vi "LSMcontroller_v66_improvedwfhandling.vi"() -> ()   [LabVIEW 2015] (continued)
                    n3096 = property on="finite samples" class="Bool (strict)"("Value"=w6474) -> ()  [unwired: 2 in, 2 out]
                    n3097 = property on="wavdet" class="Bool (strict)"("Value"=w6474) -> ()  [unwired: 2 in, 2 out]
                    n3098 = property on="save\ndata" class="Bool (strict)"("Value"=w6474) -> ()  [unwired: 2 in, 2 out]
                    n3099 = local write "Save tab"(enum32{"withsave", "withoutsave"}."withsave" ("Save tab")) -> ()
                    n3100 = property on="# of frames" class="DigNum (strict)"("DisabledEnum"=T7."Disabled and Grayed Out" ("Disabled")) -> ()  [unwired: 2 in, 2 out]
                    n3101 = property on="save\ndata" class="Bool (strict)"("DisabledEnum"=T7."Disabled and Grayed Out" ("Disabled")) -> ()  [unwired: 2 in, 2 out]
                  }
                }
              }
              frame #1 {
                n3102 = local read "finite samples"() -> (w6484:bool)
                n3103 = local read "continuous"() -> (w6483:bool)
                n3104 = local read "wavdet"() -> (w6482:bool)
                n3105 = call "2pparameters.vi"("command"="get") -> ("params out"=w6478:T10)  [unwired: 1 in]
                n3106 = Bundle By Name(cluster=w6478, "finite"=w6484, "cont"=w6483, "wavdet"=w6482) -> (w6481:T10)
                n3107 = call "2pparameters.vi"("Params in"=w6481, "command"="set") -> ()  [unwired: 1 out]
              }
            }
          }
          event "wavdet": Value Change {
            n3108 = event-data() -> ("NewVal"=w6485:bool)  [unwired: 1 in]
            n3109 = flat-sequence {
              tunnel: w6485 -> [w6486]
              frame #0 {
                n3110 = case shown="False" w6486 {
                  frame False {
                    n3111 = property on="finite samples" class="Bool (strict)"("Value"=TRUE ("finite samples for recording")) -> ()  [unwired: 2 in, 2 out]
                    n3112 = property on="continuous" class="Bool (strict)"("Value"=FALSE ("continuous")) -> ()  [unwired: 2 in, 2 out]
                    n3113 = local write "Save tab"(enum32{"withsave", "withoutsave"}."withsave" ("Save tab")) -> ()
                    n3114 = property on="save\ndata" class="Bool (strict)"("DisabledEnum"=T7."Enabled" ("Disabled")) -> ()  [unwired: 2 in, 2 out]
                    n3115 = property on="# of frames" class="DigNum (strict)"("DisabledEnum"=T7."Enabled" ("Disabled")) -> ()  [unwired: 2 in, 2 out]
                    n3116 = property on="save\ndata" class="Bool (strict)"("Value"=TRUE ("save\ndata")) -> ()  [unwired: 2 in, 2 out]
                  }
                  frame True {
                    w6495 = FALSE ("finite samples for recording")
                    n3117 = property on="finite samples" class="Bool (strict)"("Value"=w6495) -> ()  [unwired: 2 in, 2 out]
                    n3118 = property on="continuous" class="Bool (strict)"("Value"=w6495) -> ()  [unwired: 2 in, 2 out]
                    n3119 = property on="save\ndata" class="Bool (strict)"("DisabledEnum"=T7."Enabled" ("Disabled")) -> ()  [unwired: 2 in, 2 out]
                    n3120 = local write "Save tab"(enum32{"withsave", "withoutsave"}."withsave" ("Save tab")) -> ()
                    n3121 = property on="# of frames" class="DigNum (strict)"("DisabledEnum"=T7."Disabled" ("Disabled")) -> ()  [unwired: 2 in, 2 out]
                    n3122 = property on="save\ndata" class="Bool (strict)"("Value"=TRUE ("save\ndata")) -> ()  [unwired: 2 in, 2 out]
                  }
                }
              }
              frame #1 {
                n3123 = local read "finite samples"() -> (w6498:bool)
                n3124 = local read "continuous"() -> (w6499:bool)
                n3125 = local read "wavdet"() -> (w6500:bool)
                n3126 = call "2pparameters.vi"("command"="get") -> ("params out"=w6504:T10)  [unwired: 1 in]
                n3127 = Bundle By Name(cluster=w6504, "finite"=w6498, "cont"=w6499, "wavdet"=w6500) -> (w6501:T10)
                n3128 = call "2pparameters.vi"("Params in"=w6501, "command"="set") -> ()  [unwired: 1 out]
              }
            }
          }
          event "cursors": Value Change {
            n3129 = event-data() -> ()  [unwired: 1 in, 5 out]
            n3130 = case shown="True" "cursors" {
              frame False {
                n3131 = property on="img_CH1" class="IntGraph (strict)"("Active Cursor"=u32 0, "Cursor.Cursor Style"=u8 0 ("Cursor Style"), "Cursor.Cursor Point Style"=u8 0 ("Cursor Point Style")) -> ("Cursor.Cursor Position:Cursor X"=w6509:dbl, "Cursor.Cursor Position:Cursor Y"=w6510:dbl)  [unwired: 2 in, 2 out]
                n3132 = property on="img_CH2" class="IntGraph (strict)"("Active Cursor"=u32 0, "Cursor.Cursor Style"=u8 0 ("Cursor Style"), "Cursor.Cursor Point Style"=u8 0 ("Cursor Point Style")) -> ()  [unwired: 2 in, 2 out]
                n3133 = local write "cursor x [pixel]"(w6509) -> ()
                n3134 = local write "cursor y [pixel]"(w6510) -> ()
              }
              frame True {
                n3135 = stacked-sequence {
                  frame #0 {
                    n3136 = call "2pparameters.vi"("command"="get") -> ("params out"=w6525:T10)  [unwired: 1 in]
                    n3137 = Unbundle By Name(w6525) -> ("Xpixels Img"=w6526:i32, "Ypixels Img"=w6523:i32)
                    n3138 = To Double Precision Float(number=w6523) -> (double precision float=w6517:dbl)
                    n3139 = To Double Precision Float(number=w6526) -> (double precision float=w6522:dbl)
                    n3140 = Divide(x=w6517, y=2.0) -> (x/y=w6518:dbl)
                    n3141 = Divide(x=w6522, y=2.0) -> (x/y=w6520:dbl)
                    n3142 = Round To Nearest(number=w6518) -> (nearest integer value=w6516:dbl)
                    n3143 = Round To Nearest(number=w6520) -> (nearest integer value=w6519:dbl)
                    n3144 = property on="img_CH1" class="IntGraph (strict)"("Active Cursor"=u32 0, "Cursor.Cursor Style"=u8 8 ("Cursor Style"), "Cursor.Cursor Point Style"=u8 5 ("Cursor Point Style"), "Cursor.Cursor Position:Cursor X"=w6519, "Cursor.Cursor Position:Cursor Y"=w6516, "Cursor.Visible"=TRUE) -> ()  [unwired: 2 in, 2 out]
                  }
                  frame #1 {
                    n3145 = call "2pparameters.vi"("command"="get") -> ("params out"=w6545:T10)  [unwired: 1 in]
                    n3146 = call "2pparameters.vi"("command"="get") -> ("params out"=w6543:T10)  [unwired: 1 in]
                    n3147 = property on="img_CH1" class="IntGraph (strict)"("Active Cursor"=u32 0, "Cursor.Cursor Style"=u8 8 ("Cursor Style"), "Cursor.Cursor Point Style"=u8 5 ("Cursor Point Style")) -> ("Cursor.Cursor Position:Cursor X"=w6538:dbl, "Cursor.Cursor Position:Cursor Y"=w6537:dbl, "Cursor.Cursor Index"=w6560:i32, "Cursor.Cursor Plot"=w6559:i32, "Cursor.Visible"=w6530:bool)  [unwired: 2 in, 2 out]
                    "cursor x [pixel]" <- w6538
                    "cursor y [pixel]" <- w6537
                    n3148 = Unbundle By Name(w6545) -> ("Vy-max Img"=w6547:dbl, "Vy-min Img"=w6534:dbl, "Ypixels Img"=w6549:i32)
                    n3149 = Unbundle By Name(w6543) -> ("VX-max Img"=w6544:dbl, "Vx-min Img"=w6532:dbl, "Xpixels Img"=w6548:i32)
                    n3150 = Subtract(x=w6547, y=w6534) -> (x-y=w6552:dbl)
                    n3151 = Subtract(x=w6544, y=w6532) -> (x-y=w6550:dbl)
                    n3152 = local read "img_CH2"() -> (w6556:sgl[][])
                    n3153 = To Double Precision Float(number=w6548) -> (double precision float=w6551:dbl)
                    n3154 = local read "img_CH1"() -> (w6557:sgl[][])
                    n3155 = To Double Precision Float(number=w6549) -> (double precision float=w6553:dbl)
                    n3156 = Index Array(array=w6557, index (row)=w6560, index (col)=w6559) -> (element=→"value CH 1":sgl)
                    n3157 = Index Array(array=w6556, index (row)=w6560, index (col)=w6559) -> (element=→"value CH 2":sgl)
                    n3158 = Divide(x=w6550, y=w6551) -> (x/y=w6554:dbl)
                    n3159 = Divide(x=w6552, y=w6553) -> (x/y=w6555:dbl)
                    n3160 = Multiply(x=w6538, y=w6554) -> (x*y=w6533:dbl)
                    n3161 = Multiply(x=w6537, y=w6555) -> (x*y=w6536:dbl)
                    n3162 = property on="img_CH2" class="IntGraph (strict)"("Active Cursor"=u32 0, "Cursor.Cursor Style"=u8 8 ("Cursor Style"), "Cursor.Cursor Point Style"=u8 5 ("Cursor Point Style"), "Cursor.Cursor Position:Cursor X"=w6538, "Cursor.Cursor Position:Cursor Y"=w6537, "Cursor.Visible"=w6530) -> ()  [unwired: 2 in, 2 out]
                    n3163 = Add(x=w6533, y=w6532) -> (x+y=w6531:dbl)
                    n3164 = Add(x=w6536, y=w6534) -> (x+y=w6535:dbl)
                    n3165 = local write "Vx-ref"(w6531) -> ()
                    n3166 = local write "Vy-ref"(w6535) -> ()
                  }
                }
              }
            }
          }
          event "img_CH1": Cursor Move {
            n3167 = event-data() -> ("CursIdx"=w6565:i32)  [unwired: 1 in]
            n3168 = Equal To 0?(x=w6565) -> (x = 0?=w6566:bool)
            n3169 = case shown="True" w6566 {
              frame False {
              }
              frame True {
                n3170 = call "2pparameters.vi"("command"="get") -> ("params out"=w6586:T10)  [unwired: 1 in]
                n3171 = call "2pparameters.vi"("command"="get") -> ("params out"=w6588:T10)  [unwired: 1 in]
                n3172 = property on="img_CH1" class="IntGraph (strict)"("Active Cursor"=u32 0, "Cursor.Cursor Style"=u8 8 ("Cursor Style"), "Cursor.Cursor Point Style"=u8 5 ("Cursor Point Style")) -> ("Cursor.Cursor Position:Cursor X"=w6575:dbl, "Cursor.Cursor Position:Cursor Y"=w6574:dbl, "Cursor.Cursor Plot"=w6594:i32, "Cursor.Cursor Index"=w6593:i32, "Cursor.Visible"=w6567:bool)  [unwired: 2 in, 2 out]
                n3173 = Unbundle By Name(w6586) -> ("Vy-max Img"=w6584:dbl, "Vy-min Img"=w6573:dbl, "Ypixels Img"=w6582:i32)
                n3174 = Unbundle By Name(w6588) -> ("VX-max Img"=w6587:dbl, "Vx-min Img"=w6568:dbl, "Xpixels Img"=w6583:i32)
                n3175 = Subtract(x=w6584, y=w6573) -> (x-y=w6579:dbl)
                n3176 = Subtract(x=w6587, y=w6568) -> (x-y=w6581:dbl)
                n3177 = local write "cursor x [pixel]"(w6575) -> ()
                n3178 = local write "cursor y [pixel]"(w6574) -> ()
                n3179 = To Double Precision Float(number=w6583) -> (double precision float=w6580:dbl)
                n3180 = To Double Precision Float(number=w6582) -> (double precision float=w6578:dbl)
                n3181 = local read "img_CH2"() -> (w6595:sgl[][])
                n3182 = local read "img_CH1"() -> (w6598:sgl[][])
                n3183 = Index Array(array=w6595, index (row)=w6594, index (col)=w6593) -> (element=w6596:sgl)
                n3184 = Index Array(array=w6598, index (row)=w6594, index (col)=w6593) -> (element=w6597:sgl)
                n3185 = Divide(x=w6581, y=w6580) -> (x/y=w6577:dbl)
                n3186 = Divide(x=w6579, y=w6578) -> (x/y=w6576:dbl)
                n3187 = local write "value CH 2"(w6596) -> ()
                n3188 = Multiply(x=w6575, y=w6577) -> (x*y=w6570:dbl)
                n3189 = local write "value CH 1"(w6597) -> ()
                n3190 = Multiply(x=w6574, y=w6576) -> (x*y=w6572:dbl)
                n3191 = Add(x=w6570, y=w6568) -> (x+y=w6569:dbl)
                n3192 = local write "Vx-ref"(w6569) -> ()
                n3193 = Add(x=w6572, y=w6573) -> (x+y=w6571:dbl)
                n3194 = property on="img_CH2" class="IntGraph (strict)"("Active Cursor"=u32 0, "Cursor.Cursor Style"=u8 8 ("Cursor Style"), "Cursor.Cursor Point Style"=u8 5 ("Cursor Point Style"), "Cursor.Cursor Position:Cursor X"=w6575, "Cursor.Cursor Position:Cursor Y"=w6574, "Cursor.Visible"=w6567) -> ()  [unwired: 2 in, 2 out]
                n3195 = local write "Vy-ref"(w6571) -> ()
              }
            }
          }
          event "img_CH2": Cursor Move {
            n3196 = event-data() -> ("CursIdx"=w6602:i32)  [unwired: 1 in]
            n3197 = Equal To 0?(x=w6602) -> (x = 0?=w6603:bool)
            n3198 = case shown="True" w6603 {
              frame False {
              }
              frame True {
                n3199 = property on="img_CH2" class="IntGraph (strict)"("Active Cursor"=u32 0, "Cursor.Cursor Style"=u8 8 ("Cursor Style"), "Cursor.Cursor Point Style"=u8 5 ("Cursor Point Style")) -> ("Cursor.Cursor Position:Cursor X"=w6611:dbl, "Cursor.Cursor Position:Cursor Y"=w6612:dbl, "Cursor.Cursor Plot"=w6631:i32, "Cursor.Cursor Index"=w6630:i32, "Cursor.Visible"=w6604:bool)  [unwired: 2 in, 2 out]
                n3200 = call "2pparameters.vi"("command"="get") -> ("params out"=w6623:T10)  [unwired: 1 in]
                n3201 = call "2pparameters.vi"("command"="get") -> ("params out"=w6625:T10)  [unwired: 1 in]
                n3202 = local read "img_CH1"() -> (w6635:sgl[][])
                n3203 = local read "img_CH2"() -> (w6632:sgl[][])
                n3204 = local write "cursor x [pixel]"(w6611) -> ()
                n3205 = local write "cursor y [pixel]"(w6612) -> ()
                n3206 = Unbundle By Name(w6623) -> ("Vy-max Img"=w6621:dbl, "Vy-min Img"=w6606:dbl, "Ypixels Img"=w6619:i32)
                n3207 = Unbundle By Name(w6625) -> ("VX-max Img"=w6624:dbl, "Vx-min Img"=w6609:dbl, "Xpixels Img"=w6620:i32)
                n3208 = Index Array(array=w6635, index (row)=w6631, index (col)=w6630) -> (element=w6634:sgl)
                n3209 = Index Array(array=w6632, index (row)=w6631, index (col)=w6630) -> (element=w6633:sgl)
                n3210 = local write "value CH 2"(w6633) -> ()
                n3211 = local write "value CH 1"(w6634) -> ()
                n3212 = Subtract(x=w6621, y=w6606) -> (x-y=w6616:dbl)
                n3213 = Subtract(x=w6624, y=w6609) -> (x-y=w6618:dbl)
                n3214 = To Double Precision Float(number=w6620) -> (double precision float=w6617:dbl)
                n3215 = To Double Precision Float(number=w6619) -> (double precision float=w6615:dbl)
                n3216 = Divide(x=w6618, y=w6617) -> (x/y=w6614:dbl)
                n3217 = Divide(x=w6616, y=w6615) -> (x/y=w6613:dbl)
                n3218 = Multiply(x=w6611, y=w6614) -> (x*y=w6610:dbl)
                n3219 = Multiply(x=w6612, y=w6613) -> (x*y=w6607:dbl)
                n3220 = property on="img_CH1" class="IntGraph (strict)"("Active Cursor"=u32 0, "Cursor.Cursor Style"=u8 8 ("Cursor Style"), "Cursor.Cursor Point Style"=u8 5 ("Cursor Point Style"), "Cursor.Cursor Position:Cursor X"=w6611, "Cursor.Cursor Position:Cursor Y"=w6612, "Cursor.Visible"=w6604) -> ()  [unwired: 2 in, 2 out]
                n3221 = Add(x=w6610, y=w6609) -> (x+y=→"Vx-ref":dbl)
                n3222 = Add(x=w6607, y=w6606) -> (x+y=→"Vy-ref":dbl)
              }
            }
          }
          event "Focus": Value Change {
            n3223 = event-data() -> ()  [unwired: 1 in, 6 out]
            n3224 = flat-sequence {
              frame #0 {
                n3225 = local read "Focus"() -> (w6639:bool)
                n3226 = case shown="True" w6639 {
                  frame False {
                  }
                  frame True {
                    n3227 = local read "Vx-ref"() -> (w6643:dbl)
                    n3228 = local read "Vy-ref"() -> (w6642:dbl)
                    n3229 = local read "zV"() -> (w6640:dbl)
                    n3230 = call "focusvi.vi"("zc"=w6640, "yc"=w6642, "xc"=w6643) -> ("finalz"=→"zV":dbl)
                  }
                }
              }
              frame #1 {
                n3231 = local write "Focus"(FALSE ("Focus")) -> ()
              }
            }
          }
          event "auto shutter": Value Change {
            n3232 = event-data() -> ()  [unwired: 1 in, 6 out]
            n3233 = call "2pparameters.vi"("command"="get") -> ("params out"=w6647:T10)  [unwired: 1 in]
            n3234 = in-place {
              n3235 = in-place-cluster #46(w6647) -> ()  [unwired: 1 out]
              n3236 = local read "auto shutter"() -> (w6649:bool)
              n3237 = in-place-cluster #46("autoshutter"=w6649) -> (w6645:T10)
            }
            n3238 = call "2pparameters.vi"("Params in"=w6645, "command"="set") -> ()  [unwired: 1 out]
          }
          event "auto OD": Value Change {
            n3239 = event-data() -> ()  [unwired: 1 in, 6 out]
            n3240 = call "2pparameters.vi"("command"="get") -> ("params out"=w6652:T10)  [unwired: 1 in]
            n3241 = in-place {
              n3242 = in-place-cluster #47(w6652) -> ()  [unwired: 1 out]
              n3243 = local read "auto OD"() -> (w6654:bool)
              n3244 = in-place-cluster #47("auto OD"=w6654) -> (w6650:T10)
            }
            n3245 = call "2pparameters.vi"("Params in"=w6650, "command"="set") -> ()  [unwired: 1 out]
          }
          event "ODfilt": Value Change {
            n3246 = event-data() -> ("OldVal"=w6655:u16)  [unwired: 1 in, 5 out]
            n3247 = local read "ODfilt"() -> (w6656:u16)
            n3248 = call "2pparameters.vi"("command"="get") -> ("params out"=w6659:T10)  [unwired: 1 in]
            n3249 = call "filterwheelcontrol_nothorlabslib.vi"("Current OD filt"=w6655, "New ODfilt"=w6656) -> ()  [unwired: 1 in]
            n3250 = in-place {
              in-place-border: w6656 -> [w6661]
              n3251 = in-place-cluster #48(w6659) -> ()  [unwired: 1 out]
              n3252 = in-place-cluster #48("ODfilt"=w6661) -> (w6657:T10)
            }
            n3253 = call "2pparameters.vi"("Params in"=w6657, "command"="set") -> ()  [unwired: 1 out]
          }
          event "Exit": Value Change {
            n3254 = event-data() -> ()  [unwired: 1 in, 5 out]
          }
        }
        n3255 = Wait (ms)(milliseconds to wait=u32 50) -> ()  [unwired: 1 out]
      }
      n3256 = while {
        stop <- w69 stop-if-true
        # "Waveform generation"
        n3257 = event shown="[9] \"load changed AOsq\": Value Change" {
          selector: _ -> [_ _ _ _ _ _ _ _ _ _ _ _ _ _ _ _ _ _ _ _ _ _]
          dyn-events: _ -> [_ _ _ _ _ _ _ _ _ _ _ _ _ _ _ _ _ _ _ _ _ _]
          timeout: _ -> [_ _ _ _ _ _ _ _ _ _ _ _ _ _ _ _ _ _ _ _ _ _]
          tunnel: [_ _ _ _ _ _ _ _ _ _ _ _ _ _ _ _ _ _ _ _ _ w2239] -> w69
          event Timeout {
            n3258 = event-data() -> ()  [unwired: 1 in, 3 out]
          }
          event "Add AO wave": Value Change {
            n3259 = event-data() -> ("NewVal"=w70:bool)  [unwired: 1 in, 5 out]
            n3260 = case shown="True" w70 {
              frame False {
              }
              frame True {
                n3261 = stacked-sequence {
                  seq-local: [_ _ w177 _ _ _ _ _] -> [_ _ _ w209 w220 w228 w294 w326]
                  frame #0 {
                    n3262 = local read "Measurement"() -> (w71:T4)
                    n3263 = case shown="\"Timetrace\"" w71 {
                      frame "X-Y-t movie", Default {
                        n3264 = local read "avpp"() -> (w92:i32)
                        n3265 = local read "Angle ref"() -> (w91:dbl)
                        n3266 = local read "ROI Type"() -> (w90:u16)
                        n3267 = local read "xpixels ref"() -> (w87:i32)
                        n3268 = local read "Vx-min ref"() -> (w86:dbl)
                        n3269 = local read "Vx-max ref"() -> (w85:dbl)
                        n3270 = local read "ypixels ref"() -> (w83:i32)
                        n3271 = local read "Vy-min ref"() -> (w84:dbl)
                        n3272 = local read "Vy-max ref"() -> (w80:dbl)
                        n3273 = local read "Sampling rate"() -> (w74:dbl)
                        n3274 = local read "finite samples"() -> (w75:bool)
                        n3275 = local read "continuous"() -> (w78:bool)
                        n3276 = local read "wavdet"() -> (w79:bool)
                        n3277 = local read "# of frames"() -> (w77:i32)
                        n3278 = local read "maxbufferAI"() -> (w76:i32)
                        n3279 = local read "Override AI buffer"() -> (w72:bool)
                        n3280 = call "2pparameters.vi"("command"="get") -> ("params out"=w89:T10)  [unwired: 1 in]
                        n3281 = Bundle By Name(cluster=w89, "type"="X-Y-t movie", "avpp"=w92, "Angle Img"=w91, "Xpixels Img"=w87, "Vx-min Img"=w86, "VX-max Img"=w85, "Ypixels Img"=w83, "Vy-min Img"=w84, "Vy-max Img"=w80, "srate"=w74, "srate Img"=w74, "finite"=w75, "cont"=w78, "wavdet"=w79, "measpoints"=w77, "maxbufferAI"=w76, "Drawing Mode"=w90, "Vz-reset"=0.0, "AIoverride"=w72) -> (w81:T10)
                        n3282 = call "2pparameters.vi"("Params in"=w81, "command"="set") -> ()  [unwired: 1 out]
                      }
                      frame "X-Y-Z stack" {
                        n3283 = call "2pparameters.vi"("command"="get") -> ("params out"=w96:T10)  [unwired: 1 in]
                        n3284 = Bundle By Name(cluster=w96, "type"="X-Y-Z stack") -> (w94:T10)
                        n3285 = call "2pparameters.vi"("Params in"=w94, "command"="set") -> ()  [unwired: 1 out]
                      }
                      frame "Lifetime (scan)" {
                        n3286 = call "2pparameters.vi"("command"="get") -> ("params out"=w101:T10)  [unwired: 1 in]
                        n3287 = Bundle By Name(cluster=w101, "type"="Lifetime (scan)") -> (w99:T10)
                        n3288 = call "2pparameters.vi"("Params in"=w99, "command"="set") -> ()  [unwired: 1 out]
                      }
                      frame "Lifetime (contour)" {
                        n3289 = local read "Vy-min draw"() -> (w111:dbl)
                        n3290 = local read "Vy-max draw"() -> (w110:dbl)
                        n3291 = local read "Vx-min draw"() -> (w113:dbl)
                        n3292 = local read "Vx-max draw"() -> (w112:dbl)
                        n3293 = local read "xpixels ref"() -> (w109:i32)
                        n3294 = local read "ypixels ref"() -> (w108:i32)
                        n3295 = local read "ROI Type"() -> (w107:u16)
                        n3296 = local read "srateAODOtt"() -> (w118:dbl)
                        n3297 = local read "# of frames"() -> (w123:i32)
                        n3298 = local read "refreshtime"() -> (w115:dbl)
                        n3299 = local read "Pel"() -> (w106:dbl)
                        n3300 = local read "bin"() -> (w121:dbl)
                        n3301 = local read "Override AI buffer"() -> (w104:bool)
                        n3302 = local read "finite samples"() -> (w130:bool)
                        n3303 = local read "srateAODOtt"() -> (w117:dbl)
                        n3304 = local read "srateAODOtt"() -> (w124:dbl)
                        n3305 = local read "continuous"() -> (w129:bool)
                        n3306 = local read "Angle ref"() -> (w114:dbl)
                        n3307 = local read "wavdet"() -> (w131:bool)
                        n3308 = local read "Vx-ref"() -> (w126:dbl)
                        n3309 = local read "Vy-ref"() -> (w128:dbl)
                        n3310 = local read "avpp"() -> (w127:i32)
                        n3311 = call "tt_timeandsamples.vi"("bin"=w121, "refreshtime"=w115, "srateAODOtt"=w118, "tot#ofsamples"=w123) -> ("refreshrate"=w119:dbl, "refreshbuffer"=w120:i32, "timetracecycles"=w125:i32)  [unwired: 5 in]
                        n3312 = local read "bin"() -> (w122:dbl)
                        n3313 = call "2pparameters.vi"("command"="get") -> ("params out"=w134:T10)  [unwired: 1 in]
                        n3314 = Bundle By Name(cluster=w134, "Drawing Mode"=w107, "measpoints"=w123, "tt_cycles"=w125, "refreshbuffer"=w120, "refreshrate"=w119, "Vx-ref"=w126, "Vy-ref"=w128, "srate"=w117, "finite"=w130, "cont"=w129, "wavdet"=w131, "avpp"=w127, "srateAODO"=w124, "bufferAI"=w120, "bin"=w122, "Angle Img"=w114, "Vxminref"=w113, "Vxmaxref"=w112, "Vyminref"=w111, "Vymaxref"=w110, "Xpixels Img"=w109, "Ypixels Img"=w108, "Pel"=w106, "Vz-reset"=0.0, "AIoverride"=w104, "type"="Lifetime (contour)") -> (w132:T10)
                        n3315 = Reciprocal(x=w119) -> (1/x=w116:dbl)
                        n3316 = local write "refreshtime"(w116) -> ()
                        n3317 = call "2pparameters.vi"("Params in"=w132, "command"="set") -> ()  [unwired: 1 out]
                      }
                      frame "X-Y-Z-t movie" {
                      }
                      frame "linescan" {
                      }
                      frame "Timetrace" {
                        n3318 = local read "Vy-min draw"() -> (w144:dbl)
                        n3319 = local read "Vy-max draw"() -> (w143:dbl)
                        n3320 = local read "Vx-min draw"() -> (w146:dbl)
                        n3321 = local read "Vx-max draw"() -> (w145:dbl)
                        n3322 = local read "xpixels ref"() -> (w142:i32)
                        n3323 = local read "ypixels ref"() -> (w141:i32)
                        n3324 = local read "ROI Type"() -> (w140:u16)
                        n3325 = local read "srateAODOtt"() -> (w151:dbl)
                        n3326 = local read "# of frames"() -> (w156:i32)
                        n3327 = local read "refreshtime"() -> (w148:dbl)
                        n3328 = local read "Pel"() -> (w139:dbl)
                        n3329 = local read "bin"() -> (w154:dbl)
                        n3330 = local read "Override AI buffer"() -> (w137:bool)
                        n3331 = local read "finite samples"() -> (w163:bool)
                        n3332 = local read "srateAODOtt"() -> (w150:dbl)
                        n3333 = local read "srateAODOtt"() -> (w157:dbl)
                        n3334 = local read "continuous"() -> (w162:bool)
                        n3335 = local read "Angle ref"() -> (w147:dbl)
                        n3336 = local read "wavdet"() -> (w164:bool)
                        n3337 = local read "Vx-ref"() -> (w159:dbl)
                        n3338 = local read "Vy-ref"() -> (w161:dbl)
                        n3339 = local read "avpp"() -> (w160:i32)
                        n3340 = call "tt_timeandsamples.vi"("bin"=w154, "refreshtime"=w148, "srateAODOtt"=w151, "tot#ofsamples"=w156) -> ("refreshrate"=w152:dbl, "refreshbuffer"=w153:i32, "timetracecycles"=w158:i32)  [unwired: 5 in]
                        n3341 = local read "bin"() -> (w155:dbl)
                        n3342 = call "2pparameters.vi"("command"="get") -> ("params out"=w167:T10)  [unwired: 1 in]
                        n3343 = Bundle By Name(cluster=w167, "Drawing Mode"=w140, "measpoints"=w156, "tt_cycles"=w158, "refreshbuffer"=w153, "refreshrate"=w152, "Vx-ref"=w159, "Vy-ref"=w161, "srate"=w150, "finite"=w163, "cont"=w162, "wavdet"=w164, "avpp"=w160, "srateAODO"=w157, "bufferAI"=w153, "bin"=w155, "Angle Img"=w147, "Vxminref"=w146, "Vxmaxref"=w145, "Vyminref"=w144, "Vymaxref"=w143, "Xpixels Img"=w142, "Ypixels Img"=w141, "Pel"=w139, "Vz-reset"=0.0, "AIoverride"=w137, "type"="Timetrace") -> (w165:T10)
                        n3344 = Reciprocal(x=w152) -> (1/x=w149:dbl)
                        n3345 = local write "refreshtime"(w149) -> ()
                        n3346 = call "2pparameters.vi"("Params in"=w165, "command"="set") -> ()  [unwired: 1 out]
                      }
                      frame "Lifetime (point)" {
                      }
                    }
                  }
                  frame #1 {
                    w170 = FALSE ("wavdet")
                    n3347 = call "2pparameters.vi"("command"="get") -> ("params out"=w174:T10)  [unwired: 1 in]
                    n3348 = Bundle By Name(cluster=w174, "finite"=w170, "cont"=w170, "wavdet"=TRUE) -> (w171:T10)
                    n3349 = call "2pparameters.vi"("Params in"=w171, "command"="set") -> ()  [unwired: 1 out]
                  }
                  frame #2 {
                    n3350 = local read "Meastab"() -> (w201:enum32{"X-Y Image", "Linescan", "Timetrace"})
                    n3351 = property on="AO channels" class="Ring (strict)"() -> ("RingText.Text"=w176:string)  [unwired: 2 in, 2 out]
                    n3352 = property on="refwf" class="Ring (strict)"() -> ("RingText.Text"=w200:string)  [unwired: 2 in, 2 out]
                    n3353 = local read "Build analog waveform tabs"() -> (w199:enum32{"Square", "Triangle", "Matlab"})
                    n3354 = case shown="\"X-Y Image\", Default" w201 {
                      tunnel: [w207 w208] -> w198
                      frame "X-Y Image", Default {
                        n3355 = local read "Sampling rate"() -> (w207:dbl)
                      }
                      frame "Timetrace" {
                        n3356 = local read "srateAODOtt"() -> (w208:dbl)
                      }
                    }
                    n3357 = local read "Matlab waveform path"() -> (w191:path)
                    n3358 = local read "Period (ms)"() -> (w194:dbl)
                    n3359 = local read "Frequency"() -> (w193:dbl)
                    n3360 = local read "Tri Repeats"() -> (w192:dbl)
                    n3361 = local read "Repeats"() -> (w197:dbl)
                    n3362 = local read "Cycles"() -> (w196:dbl)
                    n3363 = local read "Pulses"() -> (w195:dbl)
                    n3364 = call "matlabwfexistsdialogue.vi"("Matlab waveform path"=w191) -> ("mtalab waveform path out"=w190:path)
                    n3365 = call "wfsizecalc.vi"("Sampling frequency (Hz)"=w198, "AOtab"=w199, "reference waveforms to"=w200, "channel"=w176, "Repeats"=w197, "Cycles"=w196, "Matlab wave file"=w190, "pulses"=w195, "Period (ms)"=w194, "Frequency"=w193, "Tri Repeats"=w192) -> ("total size GB"=w185:dbl, "gigabytesize wf"=w181:dbl)  [unwired: 3 in]
                    n3366 = Greater?(x=w181, y=0.5) -> (0:w182:bool)
                    n3367 = Number To Fractional String(number=w181, width (-)=i16 3) -> (F-format string=w187:string)  [unwired: 2 in]
                    n3368 = Number To Fractional String(number=w185, width (-)=i16 4) -> (F-format string=w186:string)  [unwired: 2 in]
                    n3369 = Concatenate Strings("this is a crude approximation:\nyou're about to create a  " ("message"), w187, " GB waveform for a total of " ("string"), w186, " GB. Are you sure?" ("string")) -> (w183:string)
                    n3370 = case shown="True" w182 {
                      tunnel: w183 -> [_ w206]
                      tunnel: [TRUE ("T button?") w203] -> w177
                      frame False {
                      }
                      frame True {
                        n3371 = Two Button Dialog(message=w206, 1:"No, don't do this." ("Center Button Text (\"No\")"), 2:"Yes, continue. " ("Left Button Text (\"Yes\")")) -> (T button?=w203:bool)
                      }
                    }
                  }
                  frame #3 {
                    n3372 = case shown="True" w209 {
                      frame False {
                      }
                      frame True {
                        # "change active waveform numbers array"
                        n3373 = local read "AO channels"() -> (w215:u32)
                        n3374 = call "2pparameters.vi"("command"="get") -> ("params out"=w213:T10)  [unwired: 1 in]
                        n3375 = in-place {
                          in-place-border: w215 -> [w219]
                          in-place-border: [w216] -> w210
                          n3376 = in-place-cluster #49(w213) -> ("aAO"=w218:u32[])
                          n3377 = call "add channel to active arrayv2.vi"("line array in"=w218, "line to add"=w219) -> ("line array out"=w217:u32[], "addition"=w216:bool)  [unwired: 1 out]
                          n3378 = in-place-cluster #49("aAO"=w217) -> (w211:T10)
                        }
                        n3379 = local write "addAO"(w210) -> ()
                        n3380 = call "2pparameters.vi"("Params in"=w211, "command"="set") -> ()  [unwired: 1 out]
                      }
                    }
                  }
                  frame #4 {
                    n3381 = case shown="True" w220 {
                      frame False {
                      }
                      frame True {
                        # "update GUI"
                        n3382 = local read "addAO"() -> (w221:bool)
                        n3383 = case shown="True" w221 {
                          frame False {
                          }
                          frame True {
                            n3384 = call "Used AO lines.vi"() -> ("used AO names"=w225:string[], "used AO lines"=w227:tag[])  [unwired: 2 in]
                            n3385 = control-ref of="Analog Lines Plot"() -> (w226:refnum<vi>)
                            n3386 = control-ref of="Digital Lines Plot"() -> (w224:refnum<vi>)
                            n3387 = call "Used DO lines.vi"() -> ("used DO names"=w223:string[], "used DO lines"=w222:tag[])  [unwired: 2 in]
                            n3388 = local write "Analog Used Lines"(w227) -> ()
                            n3389 = local write "Analog Used Names"(w225) -> ()
                            n3390 = local write "Digital Used Lines"(w222) -> ()
                            n3391 = local write "Digital Used Names"(w223) -> ()
                            n3392 = call "prepDOWaveplot.vi"("DigitalGraph in"=w224, "used DO names"=w223) -> ()  [unwired: 1 in]
                            n3393 = call "prepAOWaveplot.vi"("WaveformGraph in"=w226, "Analog Used Names"=w225) -> ()  [unwired: 1 in]
                          }
                        }
                      }
                    }
                  }
                  frame #5 {
                    n3394 = case shown="True" w228 {
                      frame False {
                      }
                      frame True {
                        n3395 = local read "addAO"() -> (w229:bool)
                        n3396 = case shown="True" w229 {
                          frame False {
                          }
                          frame True {
                            # "add parameters\nto parameter array"
                            n3397 = local read "Build analog waveform tabs"() -> (w230:enum32{"Square", "Triangle", "Matlab"})
                            n3398 = case shown="\"Matlab\"" w230 {
                              frame "Square", Default {
                                w243 = 0.0 ("Offset (V)")
                                n3399 = local read "Meastab"() -> (w232:enum32{"X-Y Image", "Linescan", "Timetrace"})
                                n3400 = call "waveformparamsv2.vi"("command"="get") -> ("Params out"=w241:T14)  [unwired: 4 in, 2 out]
                                n3401 = Unbundle By Name(w241) -> ("AO parameters"=w238:T15)
                                n3402 = case shown="\"Timetrace\"" w232 {
                                tunnel: [w254 w255] -> w231
                                frame "X-Y Image", Default {
                                n3403 = local read "Sampling rate"() -> (w254:dbl)
                                }
                                frame "Timetrace" {
                                n3404 = local read "srateAODOtt"() -> (w255:dbl)
                                }
                                }
                                n3405 = local read "Start amplitude (V)"() -> (w251:dbl)
                                n3406 = local read "phase shift (ms)"() -> (w244:dbl)
                                n3407 = local read "Step size (V)"() -> (w249:dbl)
                                n3408 = local read "Baseline (V)"() -> (w250:dbl)
                                n3409 = local read "Period (ms)"() -> (w247:dbl)
                                n3410 = local read "padding value"() -> (w234:dbl)
                                n3411 = local read "Repeats"() -> (w253:dbl)
                                n3412 = local read "DC (%)"() -> (w248:dbl)
                                n3413 = local read "Cycles"() -> (w252:dbl)
                                n3414 = local read "Pulses"() -> (w245:dbl)
                                n3415 = Index Array(array=w238, index=0) -> (element=w239:T16)
                                n3416 = Bundle By Name(cluster=w239, "AOtab"=0.0 ("Repeats"), "Repeats"=w253, "Cycles"=w252, "Start amplitude (V)"=w251, "Baseline (V)"=w250, "Step size (V)"=w249, "DC (%)"=w248, "Sampling frequency (Hz)"=w231, "Period (ms)"=w247, "Offset (V)"=w243, "Amplitude (V)"=w243, "Frequency"=w243, "Tri Repeats"=w243, "phase shift (ms)"=w244, "Pulses"=w245, "Matlab wave file"=path "", "padding value"=w234) -> (w236:T16)
                                n3417 = Build Array(w236) -> (w235:T15)
                                n3418 = call "waveformparamsv2.vi"("command"="add AO", "add AO"=w235) -> ()  [unwired: 3 in, 3 out]
                              }
                              frame "Matlab" {
                                w261 = 0.0 ("Repeats")
                                n3419 = local read "Meastab"() -> (w257:enum32{"X-Y Image", "Linescan", "Timetrace"})
                                n3420 = call "waveformparamsv2.vi"("command"="get") -> ("Params out"=w268:T14)  [unwired: 4 in, 2 out]
                                n3421 = Unbundle By Name(w268) -> ("AO parameters"=w265:T15)
                                n3422 = case shown="\"Timetrace\"" w257 {
                                tunnel: [w271 w272] -> w256
                                frame "X-Y Image", Default {
                                n3423 = local read "Sampling rate"() -> (w271:dbl)
                                }
                                frame "Timetrace" {
                                n3424 = local read "srateAODOtt"() -> (w272:dbl)
                                }
                                }
                                n3425 = local read "Matlab waveform path"() -> (w258:path)
                                n3426 = local read "Matlab padding value"() -> (w260:dbl)
                                n3427 = Index Array(array=w265, index=0) -> (element=w266:T16)
                                n3428 = call "matlabwfexistsdialogue.vi"("Matlab waveform path"=w258) -> ("mtalab waveform path out"=w259:path)
                                n3429 = Bundle By Name(cluster=w266, "AOtab"=2.0 ("Repeats"), "Repeats"=w261, "Cycles"=w261, "Start amplitude (V)"=w261, "Baseline (V)"=w261, "Step size (V)"=w261, "DC (%)"=w261, "Sampling frequency (Hz)"=w256, "Period (ms)"=w261, "Offset (V)"=w261, "Amplitude (V)"=w261, "Frequency"=w261, "Tri Repeats"=w261, "phase shift (ms)"=w261, "Pulses"=w261, "Matlab wave file"=w259, "padding value"=w260) -> (w263:T16)
                                n3430 = Build Array(w263) -> (w262:T15)
                                n3431 = call "waveformparamsv2.vi"("command"="add AO", "add AO"=w262) -> ()  [unwired: 3 in, 3 out]
                              }
                              frame "Triangle" {
                                w278 = 0.0 ("Offset (V)")
                                n3432 = local read "Meastab"() -> (w274:enum32{"X-Y Image", "Linescan", "Timetrace"})
                                n3433 = call "waveformparamsv2.vi"("command"="get") -> ("Params out"=w290:T14)  [unwired: 4 in, 2 out]
                                n3434 = Unbundle By Name(w290) -> ("AO parameters"=w287:T15)
                                n3435 = case shown="\"Timetrace\"" w274 {
                                tunnel: [w292 w293] -> w273
                                frame "X-Y Image", Default {
                                n3436 = local read "Sampling rate"() -> (w292:dbl)
                                }
                                frame "Timetrace" {
                                n3437 = local read "srateAODOtt"() -> (w293:dbl)
                                }
                                }
                                n3438 = local read "Tri padding value"() -> (w276:dbl)
                                n3439 = local read "Amplitude (V)"() -> (w281:dbl)
                                n3440 = local read "Tri Phase (s)"() -> (w277:dbl)
                                n3441 = local read "Tri Repeats"() -> (w279:dbl)
                                n3442 = local read "Frequency"() -> (w280:dbl)
                                n3443 = local read "Offset (V)"() -> (w282:dbl)
                                n3444 = Index Array(array=w287, index=0) -> (element=w288:T16)
                                n3445 = Bundle By Name(cluster=w288, "AOtab"=1.0 ("Repeats"), "Repeats"=w278, "Cycles"=w278, "Start amplitude (V)"=w278, "Baseline (V)"=w278, "Step size (V)"=w278, "DC (%)"=w278, "Sampling frequency (Hz)"=w273, "Period (ms)"=w278, "Offset (V)"=w282, "Amplitude (V)"=w281, "Frequency"=w280, "Tri Repeats"=w279, "phase shift (ms)"=w278, "Pulses"=w278, "Matlab wave file"=path "", "Tri phase"=w277, "padding value"=w276) -> (w285:T16)
                                n3446 = Build Array(w285) -> (w284:T15)
                                n3447 = call "waveformparamsv2.vi"("command"="add AO", "add AO"=w284) -> ()  [unwired: 3 in, 3 out]
                              }
                            }
                          }
                        }
                      }
                    }
                  }
                  frame #6 {
                    n3448 = case shown="True" w294 {
                      frame False {
                      }
                      frame True {
                        n3449 = local read "addAO"() -> (w295:bool)
                        n3450 = case shown="True" w295 {
                          frame False {
                          }
                          frame True {
                            # "add waveform to waveform array; correct waveform lengths and plot"
                            n3451 = local read "Meastab"() -> (w299:enum32{"X-Y Image", "Linescan", "Timetrace"})
                            n3452 = local read "Build analog waveform tabs"() -> (w309:enum32{"Square", "Triangle", "Matlab"})
                            n3453 = case shown="\"Timetrace\"" w299 {
                              tunnel: [w317 w318] -> w298
                              frame "X-Y Image", Default {
                                n3454 = local read "Sampling rate"() -> (w317:dbl)
                              }
                              frame "Timetrace" {
                                n3455 = local read "srateAODOtt"() -> (w318:dbl)
                              }
                            }
                            n3456 = call "waveformparamsv2.vi"("command"="get last AO") -> ("last AO"=w311:T16)  [unwired: 4 in, 2 out]
                            n3457 = case shown="\"Square\", Default" w309 {
                              tunnel: w311 -> [w321 w323 w325]
                              tunnel: [w320 w322 w324] -> w310
                              frame "Square", Default {
                                n3458 = call "generateRampedSquareWave_fromAOparameters.vi"("AO params"=w321) -> ("Waveform"=w320:waveform(dbl))  [unwired: 1 out]
                              }
                              frame "Triangle" {
                                n3459 = call "generateTriWave_fromAOparameters.vi"("AO params"=w323) -> ("Waveform"=w322:waveform(dbl))  [unwired: 1 out]
                              }
                              frame "Matlab" {
                                n3460 = call "matlabAOwffromparam.vi"("Cluster"=w325) -> ("Waveform"=w324:waveform(dbl))  [unwired: 1 out]
                              }
                            }
                            n3461 = property on="refwf" class="Ring (strict)"() -> ("RingText.Text"=w302:string)  [unwired: 2 in, 2 out]
                            n3462 = call "waveformsAObuffer.vi"("command"="get") -> ("AO wf out"=w315:waveform(dbl)[])  [unwired: 1 in]
                            n3463 = Build Array (concatenate)(w315, w310) -> (w312:waveform(dbl)[])
                            n3464 = call "waveformsDObuffer.vi"("command"="get") -> ("DO wf out"=w307:digitalwaveform[])  [unwired: 1 in]
                            n3465 = call "correctwaveformsizetemp.vi"("new sampling frequency (Hz)"=w298, "start"=FALSE, "reference waveforms to"=w302, "Analog waveforms in"=w312, "stop"=FALSE, "Digital waveforms in"=w307) -> ("analog wf out"=w305:waveform(dbl)[], "Digital wf out"=w303:digitalwaveform[], "measpoints"=w300:i32)
                            n3466 = local write "Analog Lines Plot"(w305) -> ()
                            n3467 = call "GetNumCamFramesv2.vi"("Digital Waveform Graph"=w303) -> ("Numeric"=w304:i32)  [unwired: 10 in]
                            n3468 = local write "Digital Lines Plot"(w303) -> ()
                            n3469 = call "waveformsAObuffer.vi"("AO wf in"=w305, "command"="set") -> ()  [unwired: 1 out]
                            n3470 = call "waveformsDObuffer.vi"("DO wf in"=w303, "command"="set") -> ()  [unwired: 1 out]
                            n3471 = local write "Total Camera Frames"(w304) -> ()
                            n3472 = local read "wavdet"() -> (w301:bool)
                            n3473 = case shown="True" w301 {
                              tunnel: w300 -> [_ w319]
                              frame False {
                              }
                              frame True {
                                n3474 = local write "# of frames"(w319) -> ()
                              }
                            }
                          }
                        }
                      }
                    }
                  }
                  frame #7 {
                    w327 = FALSE ("addAO")
                    # "set signaling boolean to false"
                    n3475 = case shown="True" w326 {
                      frame False {
                      }
                      frame True {
                        n3476 = local read "Build analog waveform tabs"() -> (w335:enum32{"Square", "Triangle", "Matlab"})
                        n3477 = case shown="\"Triangle\"" w335 {
                          frame "Square", Default {
                            n3478 = local write "not loaded"(FALSE ("not loaded")) -> ()
                          }
                          frame "Triangle" {
                            n3479 = local write "not loadedtri"(FALSE ("not loadedtri")) -> ()
                          }
                          frame "Matlab" {
                            n3480 = local write "not loadedml"(FALSE ("not loadedml")) -> ()
                          }
                        }
                      }
                    }
                    n3481 = local read "finite samples"() -> (w328:bool)
                    n3482 = local read "continuous"() -> (w329:bool)
                    n3483 = local read "wavdet"() -> (w330:bool)
                    n3484 = call "2pparameters.vi"("command"="get") -> ("params out"=w333:T10)  [unwired: 1 in]
                    n3485 = Bundle By Name(cluster=w333, "finite"=w328, "cont"=w329, "wavdet"=w330) -> (w331:T10)
                    n3486 = local write "addAO"(w327) -> ()
                    n3487 = property on="Add AO wave" class="Bool (strict)"("Val(Sgnl)"=w327) -> ()  [unwired: 2 in, 2 out]
                    n3488 = call "2pparameters.vi"("Params in"=w331, "command"="set") -> ()  [unwired: 1 out]
                  }
                }
              }
            }
          }
          event "AO channels": Value Change {
            n3489 = event-data() -> ()  [unwired: 1 in, 6 out]
            n3490 = local read "AO channels"() -> (w339:u32)
            n3491 = call "2pparameters.vi"("command"="get") -> ("params out"=w341:T10)  [unwired: 1 in]
            n3492 = Unbundle By Name(w341) -> ("aAO"=w340:u32[])
            n3493 = Search 1D Array(1D array=w340, element=w339) -> (index of element=w343:i32)  [unwired: 1 in]
            n3494 = Equal?(x=w343, y=-1.0) -> (x = y?=w344:bool)
            n3495 = case shown="False" w344 {
              tunnel: w343 -> [w346 _]
              frame False {
                n3496 = call "waveformparamsv2.vi"("command"="get") -> ("Params out"=w353:T14)  [unwired: 4 in, 2 out]
                n3497 = Unbundle By Name(w353) -> ("AO parameters"=w352:T15)
                n3498 = Index Array(array=w352, index=w346) -> (element=w369:T16)
                n3499 = Unbundle By Name(w369) -> ("AOtab"=w350:dbl, "Repeats"=w368:dbl, "Cycles"=w367:dbl, "Start amplitude (V)"=w366:dbl, "Baseline (V)"=w365:dbl, "Step size (V)"=w364:dbl, "DC (%)"=w363:dbl, "Sampling frequency (Hz)"=w362:dbl, "Period (ms)"=w361:dbl, "Offset (V)"=w360:dbl, "Amplitude (V)"=w359:dbl, "Frequency"=w358:dbl, "Tri Repeats"=w357:dbl, "phase shift (ms)"=w356:dbl, "Pulses"=w355:dbl, "Tri phase"=w351:dbl, "padding value"=w347:dbl, "Matlab wave file"=w348:path)
                n3500 = To Unsigned Long Integer(number=w350) -> (unsigned 32bit integer=w349:u32)
                n3501 = local write "Build analog waveform tabs"(w349) -> ()
                n3502 = local write "Matlab waveform path"(w348) -> ()
                n3503 = local write "phase shift (ms)"(w356) -> ()
                n3504 = local write "Repeats"(w368) -> ()
                n3505 = local write "Cycles"(w367) -> ()
                n3506 = local write "Amplitude (V)"(w359) -> ()
                n3507 = local write "Matlab padding value"(w347) -> ()
                n3508 = local write "Tri padding value"(w347) -> ()
                n3509 = local write "Start amplitude (V)"(w366) -> ()
                n3510 = local write "Tri Phase (s)"(w351) -> ()
                n3511 = local write "Period (ms)"(w361) -> ()
                n3512 = local write "Tri Repeats"(w357) -> ()
                n3513 = local write "Offset (V)"(w360) -> ()
                n3514 = local write "Frequency"(w358) -> ()
                n3515 = local write "Pulses"(w355) -> ()
                n3516 = local write "padding value"(w347) -> ()
                n3517 = local write "Sampling rate \ncurrent wf"(w362) -> ()
                n3518 = local write "Baseline (V)"(w365) -> ()
                n3519 = local write "Step size (V)"(w364) -> ()
                n3520 = local write "DC (%)"(w363) -> ()
              }
              frame True {
              }
            }
          }
          event "Rem AO wave": Value Change {
            n3521 = event-data() -> ("NewVal"=w370:bool)  [unwired: 1 in, 5 out]
            n3522 = case shown="True" w370 {
              frame False {
              }
              frame True {
                n3523 = stacked-sequence {
                  seq-local: [_ _ w476 _ _ _ _] -> [_ _ _ _ w496 w499 _]
                  frame #0 {
                    n3524 = local read "Measurement"() -> (w371:T4)
                    n3525 = case shown="\"X-Y-t movie\", Default" w371 {
                      frame "X-Y-t movie", Default {
                        n3526 = local read "avpp"() -> (w392:i32)
                        n3527 = local read "Angle ref"() -> (w391:dbl)
                        n3528 = local read "ROI Type"() -> (w390:u16)
                        n3529 = local read "xpixels ref"() -> (w387:i32)
                        n3530 = local read "Vx-min ref"() -> (w386:dbl)
                        n3531 = local read "Vx-max ref"() -> (w385:dbl)
                        n3532 = local read "ypixels ref"() -> (w383:i32)
                        n3533 = local read "Vy-min ref"() -> (w384:dbl)
                        n3534 = local read "Vy-max ref"() -> (w380:dbl)
                        n3535 = local read "Sampling rate"() -> (w374:dbl)
                        n3536 = local read "finite samples"() -> (w375:bool)
                        n3537 = local read "continuous"() -> (w378:bool)
                        n3538 = local read "wavdet"() -> (w379:bool)
                        n3539 = local read "# of frames"() -> (w377:i32)
                        n3540 = local read "maxbufferAI"() -> (w376:i32)
                        n3541 = local read "Override AI buffer"() -> (w372:bool)
                        n3542 = call "2pparameters.vi"("command"="get") -> ("params out"=w389:T10)  [unwired: 1 in]
                        n3543 = Bundle By Name(cluster=w389, "type"="X-Y-t movie", "avpp"=w392, "Angle Img"=w391, "Xpixels Img"=w387, "Vx-min Img"=w386, "VX-max Img"=w385, "Ypixels Img"=w383, "Vy-min Img"=w384, "Vy-max Img"=w380, "srate"=w374, "srate Img"=w374, "finite"=w375, "cont"=w378, "wavdet"=w379, "measpoints"=w377, "maxbufferAI"=w376, "Drawing Mode"=w390, "Vz-reset"=0.0, "AIoverride"=w372) -> (w381:T10)
                        n3544 = call "2pparameters.vi"("Params in"=w381, "command"="set") -> ()  [unwired: 1 out]
                      }
                      frame "X-Y-Z stack" {
                        n3545 = call "2pparameters.vi"("command"="get") -> ("params out"=w396:T10)  [unwired: 1 in]
                        n3546 = Bundle By Name(cluster=w396, "type"="X-Y-Z stack") -> (w394:T10)
                        n3547 = call "2pparameters.vi"("Params in"=w394, "command"="set") -> ()  [unwired: 1 out]
                      }
                      frame "Lifetime (scan)" {
                        n3548 = call "2pparameters.vi"("command"="get") -> ("params out"=w401:T10)  [unwired: 1 in]
                        n3549 = Bundle By Name(cluster=w401, "type"="Lifetime (scan)") -> (w399:T10)
                        n3550 = call "2pparameters.vi"("Params in"=w399, "command"="set") -> ()  [unwired: 1 out]
                      }
                      frame "Lifetime (contour)" {
                        n3551 = local read "Vy-min draw"() -> (w411:dbl)
                        n3552 = local read "Vy-max draw"() -> (w410:dbl)
                        n3553 = local read "Vx-min draw"() -> (w413:dbl)
                        n3554 = local read "Vx-max draw"() -> (w412:dbl)
                        n3555 = local read "xpixels ref"() -> (w409:i32)
                        n3556 = local read "ypixels ref"() -> (w408:i32)
                        n3557 = local read "ROI Type"() -> (w407:u16)
                        n3558 = local read "srateAODOtt"() -> (w418:dbl)
                        n3559 = local read "# of frames"() -> (w423:i32)
                        n3560 = local read "refreshtime"() -> (w415:dbl)
                        n3561 = local read "Pel"() -> (w406:dbl)
                        n3562 = local read "bin"() -> (w421:dbl)
                        n3563 = local read "Override AI buffer"() -> (w404:bool)
                        n3564 = local read "finite samples"() -> (w430:bool)
                        n3565 = local read "srateAODOtt"() -> (w417:dbl)
                        n3566 = local read "srateAODOtt"() -> (w424:dbl)
                        n3567 = local read "continuous"() -> (w429:bool)
                        n3568 = local read "Angle ref"() -> (w414:dbl)
                        n3569 = local read "wavdet"() -> (w431:bool)
                        n3570 = local read "Vx-ref"() -> (w426:dbl)
                        n3571 = local read "Vy-ref"() -> (w428:dbl)
                        n3572 = local read "avpp"() -> (w427:i32)
                        n3573 = call "tt_timeandsamples.vi"("bin"=w421, "refreshtime"=w415, "srateAODOtt"=w418, "tot#ofsamples"=w423) -> ("refreshrate"=w419:dbl, "refreshbuffer"=w420:i32, "timetracecycles"=w425:i32)  [unwired: 5 in]
                        n3574 = local read "bin"() -> (w422:dbl)
                        n3575 = call "2pparameters.vi"("command"="get") -> ("params out"=w434:T10)  [unwired: 1 in]
                        n3576 = Bundle By Name(cluster=w434, "Drawing Mode"=w407, "measpoints"=w423, "tt_cycles"=w425, "refreshbuffer"=w420, "refreshrate"=w419, "Vx-ref"=w426, "Vy-ref"=w428, "srate"=w417, "finite"=w430, "cont"=w429, "wavdet"=w431, "avpp"=w427, "srateAODO"=w424, "bufferAI"=w420, "bin"=w422, "Angle Img"=w414, "Vxminref"=w413, "Vxmaxref"=w412, "Vyminref"=w411, "Vymaxref"=w410, "Xpixels Img"=w409, "Ypixels Img"=w408, "Pel"=w406, "Vz-reset"=0.0, "AIoverride"=w404, "type"="Lifetime (contour)") -> (w432:T10)
                        n3577 = Reciprocal(x=w419) -> (1/x=w416:dbl)
                        n3578 = local write "refreshtime"(w416) -> ()
                        n3579 = call "2pparameters.vi"("Params in"=w432, "command"="set") -> ()  [unwired: 1 out]
                      }
                      frame "X-Y-Z-t movie" {
                      }
                      frame "linescan" {
                      }
                      frame "Timetrace" {
                        n3580 = local read "Vy-min draw"() -> (w444:dbl)
                        n3581 = local read "Vy-max draw"() -> (w443:dbl)
                        n3582 = local read "Vx-min draw"() -> (w446:dbl)
                        n3583 = local read "Vx-max draw"() -> (w445:dbl)
                        n3584 = local read "xpixels ref"() -> (w442:i32)
                        n3585 = local read "ypixels ref"() -> (w441:i32)
                        n3586 = local read "ROI Type"() -> (w440:u16)
                        n3587 = local read "srateAODOtt"() -> (w451:dbl)
                        n3588 = local read "# of frames"() -> (w456:i32)
                        n3589 = local read "refreshtime"() -> (w448:dbl)
                        n3590 = local read "Pel"() -> (w439:dbl)
                        n3591 = local read "bin"() -> (w454:dbl)
                        n3592 = local read "Override AI buffer"() -> (w437:bool)
                        n3593 = local read "finite samples"() -> (w463:bool)
                        n3594 = local read "srateAODOtt"() -> (w450:dbl)
                        n3595 = local read "srateAODOtt"() -> (w457:dbl)
                        n3596 = local read "continuous"() -> (w462:bool)
                        n3597 = local read "Angle ref"() -> (w447:dbl)
                        n3598 = local read "wavdet"() -> (w464:bool)
                        n3599 = local read "Vx-ref"() -> (w459:dbl)
                        n3600 = local read "Vy-ref"() -> (w461:dbl)
                        n3601 = local read "avpp"() -> (w460:i32)
                        n3602 = call "tt_timeandsamples.vi"("bin"=w454, "refreshtime"=w448, "srateAODOtt"=w451, "tot#ofsamples"=w456) -> ("refreshrate"=w452:dbl, "refreshbuffer"=w453:i32, "timetracecycles"=w458:i32)  [unwired: 5 in]
                        n3603 = local read "bin"() -> (w455:dbl)
                        n3604 = call "2pparameters.vi"("command"="get") -> ("params out"=w467:T10)  [unwired: 1 in]
                        n3605 = Bundle By Name(cluster=w467, "Drawing Mode"=w440, "measpoints"=w456, "tt_cycles"=w458, "refreshbuffer"=w453, "refreshrate"=w452, "Vx-ref"=w459, "Vy-ref"=w461, "srate"=w450, "finite"=w463, "cont"=w462, "wavdet"=w464, "avpp"=w460, "srateAODO"=w457, "bufferAI"=w453, "bin"=w455, "Angle Img"=w447, "Vxminref"=w446, "Vxmaxref"=w445, "Vyminref"=w444, "Vymaxref"=w443, "Xpixels Img"=w442, "Ypixels Img"=w441, "Pel"=w439, "Vz-reset"=0.0, "AIoverride"=w437, "type"="Timetrace") -> (w465:T10)
                        n3606 = Reciprocal(x=w452) -> (1/x=w449:dbl)
                        n3607 = local write "refreshtime"(w449) -> ()
                        n3608 = call "2pparameters.vi"("Params in"=w465, "command"="set") -> ()  [unwired: 1 out]
                      }
                      frame "Lifetime (point)" {
                      }
                    }
                  }
                  frame #1 {
                    w470 = FALSE ("wavdet")
                    n3609 = call "2pparameters.vi"("command"="get") -> ("params out"=w474:T10)  [unwired: 1 in]
                    n3610 = Bundle By Name(cluster=w474, "finite"=w470, "cont"=w470, "wavdet"=TRUE) -> (w471:T10)
                    n3611 = call "2pparameters.vi"("Params in"=w471, "command"="set") -> ()  [unwired: 1 out]
                  }
                  frame #2 {
                    # "remove channel from numbers array"
                    n3612 = local read "AO channels"() -> (w481:u32)
                    n3613 = call "2pparameters.vi"("command"="get") -> ("params out"=w479:T10)  [unwired: 1 in]
                    n3614 = in-place {
                      in-place-border: w481 -> [w487]
                      in-place-border: [w484] -> w482
                      in-place-border: [w483] -> w476
                      n3615 = in-place-cluster #50(w479) -> ("aAO"=w486:u32[])
                      n3616 = call "remove channel from active arrayv2.vi"("line array in"=w486, "line to remove"=w487) -> ("line array out"=w485:u32[], "removal"=w484:bool, "index"=w483:i32)
                      n3617 = in-place-cluster #50("aAO"=w485) -> (w477:T10)
                    }
                    n3618 = local write "remAO"(w482) -> ()
                    n3619 = call "2pparameters.vi"("Params in"=w477, "command"="set") -> ()  [unwired: 1 out]
                  }
                  frame #3 {
                    n3620 = local read "remAO"() -> (w488:bool)
                    n3621 = case shown="True" w488 {
                      frame False {
                      }
                      frame True {
                        n3622 = call "Used AO lines.vi"() -> ("used AO names"=w492:string[], "used AO lines"=w494:tag[])  [unwired: 2 in]
                        n3623 = control-ref of="Analog Lines Plot"() -> (w493:refnum<vi>)
                        n3624 = control-ref of="Digital Lines Plot"() -> (w491:refnum<vi>)
                        n3625 = call "Used DO lines.vi"() -> ("used DO names"=w490:string[], "used DO lines"=w489:tag[])  [unwired: 2 in]
                        n3626 = local write "Analog Used Lines"(w494) -> ()
                        n3627 = local write "Analog Used Names"(w492) -> ()
                        n3628 = local write "Digital Used Lines"(w489) -> ()
                        n3629 = local write "Digital Used Names"(w490) -> ()
                        n3630 = call "prepDOWaveplot.vi"("DigitalGraph in"=w491, "used DO names"=w490) -> ()  [unwired: 1 in]
                        n3631 = call "prepAOWaveplot.vi"("WaveformGraph in"=w493, "Analog Used Names"=w492) -> ()  [unwired: 1 in]
                      }
                    }
                  }
                  frame #4 {
                    n3632 = local read "remAO"() -> (w495:bool)
                    n3633 = case shown="True" w495 {
                      tunnel: w496 -> [_ w497]
                      frame False {
                      }
                      frame True {
                        n3634 = call "waveformparamsv2.vi"("command"="rem AO", "index"=w497) -> ()  [unwired: 3 in, 3 out]
                      }
                    }
                  }
                  frame #5 {
                    n3635 = local read "remAO"() -> (w500:bool)
                    n3636 = case shown="True" w500 {
                      tunnel: w499 -> [_ w519]
                      frame False {
                      }
                      frame True {
                        n3637 = local read "Meastab"() -> (w504:enum32{"X-Y Image", "Linescan", "Timetrace"})
                        n3638 = property on="refwf" class="Ring (strict)"() -> ("RingText.Text"=w507:string)  [unwired: 2 in, 2 out]
                        n3639 = case shown="\"Timetrace\"" w504 {
                          tunnel: [w520 w521] -> w503
                          frame "X-Y Image", Default {
                            n3640 = local read "Sampling rate"() -> (w520:dbl)
                          }
                          frame "Timetrace" {
                            n3641 = local read "srateAODOtt"() -> (w521:dbl)
                          }
                        }
